vi "XNET SESSION START.vi"(5 "interface":refnum<k21>) -> (0 "Read":refnum<k21>, 1 "error out":errorcluster, 2 "Write":refnum<k21>)   [LabVIEW 2023]
uses:
  <vilib>/xnet/xnet.llb/XNET Create Session (Frame Input Stream).vi
  Sub VIs/Global .vi
  <vilib>/xnet/xnet.llb/XNET Create Session (Frame Output Queued).vi
  <resource>/objmgr/xnet.rc
panel:
  in  "error in (no error) 2":errorcluster
  in  "error in (no error)":errorcluster
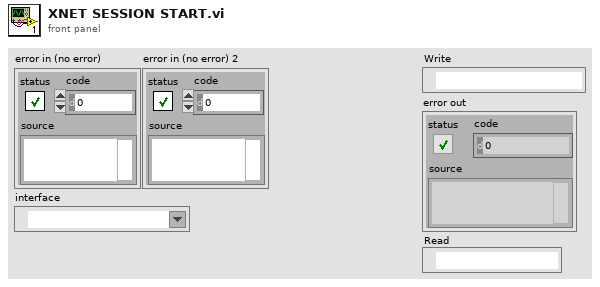
[diagram p1: front panel]
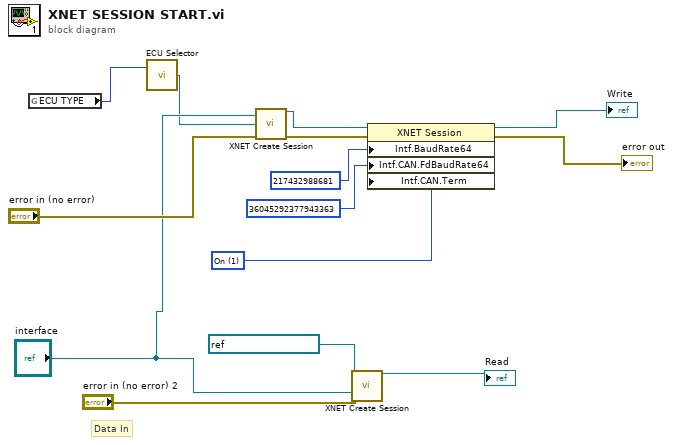
[diagram p0: block diagram]
diagram:
  w10 = u32 1 items=["Off", "On"] ("Interface:CAN:Termination")
  # "Data In"
  n1 = global read "Global .vi" "ECU TYPE"() -> (w1:u16)
  n2 = call "ECU Selector.vi"("ECU TYPE"=w1) -> ("frame"=w2:refnum<k21>)  [unwired: 1 in, 4 out]
  n3 = call-poly <vilib>:"XNET Create Session.vi"("frame"=w2, "interface"="interface", "error in (no error)"="error in (no error)") -> ("session out"=w7:refnum<k21>, "error out"=w14:errorcluster)  [unwired: 11 in]
  n4 = call-poly <vilib>:"XNET Create Session.vi"("cluster (:memory:)"=refnum<k21> "Elatch Database", "interface"="interface", "error in (no error)"="error in (no error) 2") -> ("session out"=→"Read":refnum<k21>)  [unwired: 11 in, 1 out]
  n5 = property class="XNET Session"(reference=w7, error in=w14, "Intf.BaudRate64"=u64 217432988681 ("Interface:64bit Baud Rate"), "Intf.CAN.FdBaudRate64"=u64 36045292377943363 ("Interface:CAN:64bit FD Baud Rate"), "Intf.CAN.Term"=w10) -> (reference out=→"Write":refnum<k21>, error out=→"error out":errorcluster)
